vi "FK 5-bar Mechanism.vi"(3 "error in (no error)":errorcluster, 4 "motors angles":dbl[](array[numeric])=[0.0, 0.0, 0.0, 0.0, 0.0, 0.0, 0.0], 5 "Finger in":refnum<class "Finger.lvclass">) -> (0 "error out":errorcluster, 1 "joint angles":dbl[](array[numeric]), 2 "Finger out":refnum<class "Finger.lvclass">)   [LabVIEW 2013, in "Finger.lvclass"]
uses:
  Finger.lvclass
  Finger.lvclass/Finger.ctl
panel:
  out "alpha":dbl
  out "theta":dbl
  out "psi":dbl
  out "phi":dbl
  out "d":dbl
  out "L4":dbl
  out "L3":dbl
  out "L2":dbl
  out "L1":dbl
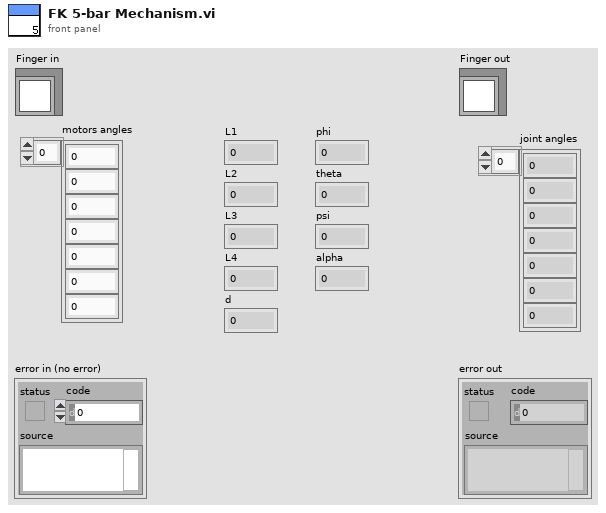
[diagram p1: front panel]
types:
  T1 = typedef "5-bar Side.ctl" = enum16{"Left", "Right"}
  T2 = cluster{"L1":dbl, "L2":dbl, "L3":dbl, "L4":dbl, "d":dbl, "d6":dbl}
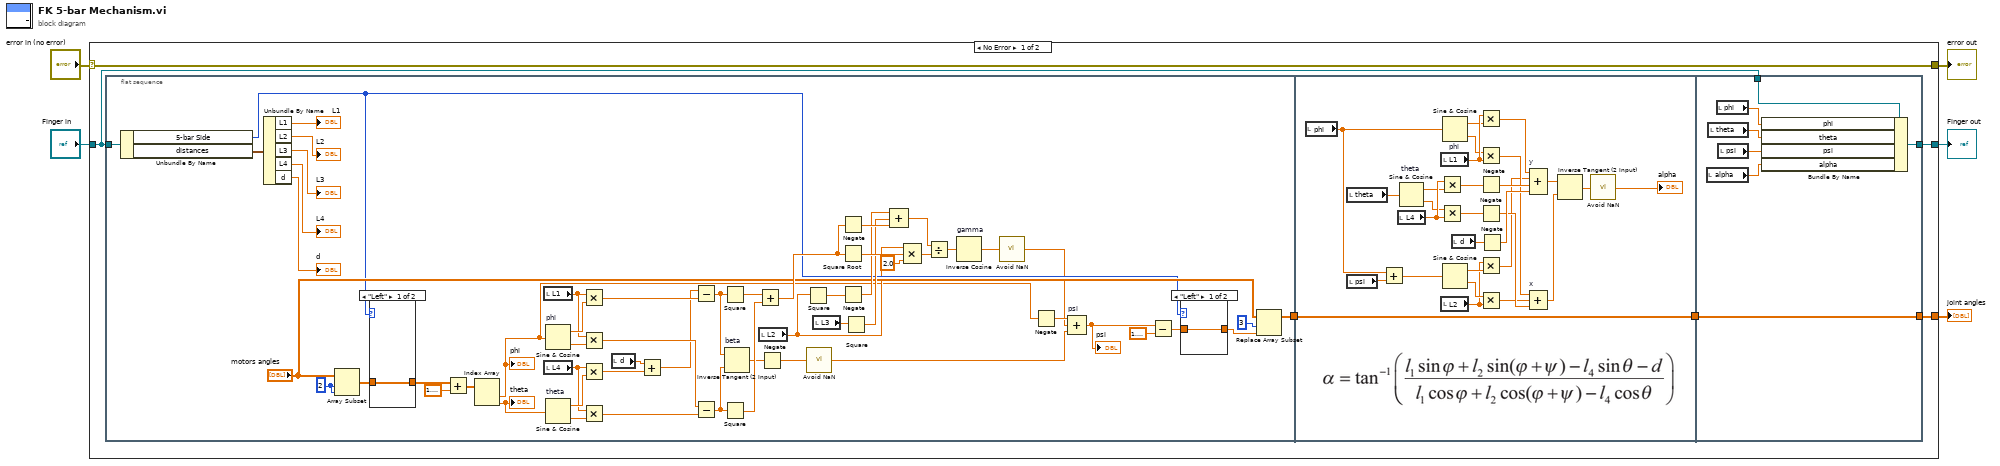
[diagram p0: block diagram]
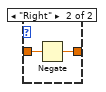
[diagram p2: hidden frame]
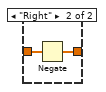
[diagram p3: hidden frame]
diagram:
  n1 = case shown="No Error" "error in (no error)" {
    selector: "error in (no error)" -> [w11 w110]
    tunnel: [w11 w110] -> w4
    tunnel: "Finger in" -> [w6 w109]
    tunnel: [w7 w109] -> w2
    tunnel: [w10 _] -> w1
    frame No Error {
      n2 = flat-sequence {
        tunnel: w6 -> [w31]
        tunnel: [w17] -> w9
        tunnel: w9 -> [w101]
        tunnel: [w101] -> w8
        tunnel: [w108] -> w10
        tunnel: w8 -> [w108]
        tunnel: [w103] -> w7
        tunnel: w6 -> [w102]
        frame #0 {
          w66 = 2 ("index")
          n3 = Unbundle By Name(w31) -> ("5-bar Side"=w30:T1, "distances"=w33:T2)
          n4 = Unbundle By Name(w33) -> ("L1"=→"L1":dbl, "L2"=→"L2":dbl, "L3"=→"L3":dbl, "L4"=→"L4":dbl, "d"=→"d":dbl)
          n5 = Array Subset(array="motors angles", index=w66, length=w66) -> (w35:dbl[])
          n6 = case shown="\"Left\"" w30 {
            tunnel: w35 -> [w71 w73]
            tunnel: [w71 w72] -> w34
            frame "Left" {
            }
            frame "Right" {
              n7 = Negate(x=w73) -> (-x=w72:dbl[])
            }
          }
          n8 = Add(x=w34, y=1.5707963267948966) -> (x+y=w36:dbl[])
          n9 = Index Array(array=w36) -> (element #1=w18:dbl, element #2=w19:dbl)  [unwired: 2 in]
          "phi" <- w18
          "theta" <- w19
          n10 = local read "L1"() -> (w27:dbl)
          n11 = local read "L4"() -> (w24:dbl)
          n12 = Sine & Cosine "phi"(0:w18) -> (1:w29:dbl, 2:w63:dbl)
          n13 = Sine & Cosine "theta"(0:w19) -> (1:w65:dbl, 2:w64:dbl)
          n14 = Multiply(x=w27, y=w29) -> (x*y=w42:dbl)
          n15 = Multiply(x=w27, y=w63) -> (x*y=w61:dbl)
          n16 = Multiply(x=w24, y=w65) -> (x*y=w41:dbl)
          n17 = Multiply(x=w24, y=w64) -> (x*y=w62:dbl)
          n18 = local read "d"() -> (w23:dbl)
          n19 = Add(x=w23, y=w41) -> (x+y=w40:dbl)
          n20 = Subtract(x=w40, y=w42) -> (x-y=w44:dbl)
          n21 = Subtract(x=w61, y=w62) -> (x-y=w43:dbl)
          n22 = Square(x=w44) -> (x^2=w60:dbl)
          n23 = Square(x=w43) -> (x^2=w59:dbl)
          n24 = Inverse Tangent (2 Input) "beta"(1:w43, 2:w44) -> (0:w48:dbl)
          n25 = Add(x=w60, y=w59) -> (x+y=w55:dbl)
          n26 = local read "L2"() -> (w28:dbl)
          n27 = Negate(x=w48) -> (-x=w16:dbl)
          n28 = Square(x=w28) -> (x^2=w57:dbl)
          n29 = call "Avoid NaN.vi"("Value"=w16) -> ("Number"=w15:dbl)
          n30 = local read "L3"() -> (w25:dbl)
          n31 = Negate(x=w55) -> (-x=w58:dbl)
          n32 = Square Root(x=w55) -> (sqrt(x)=w54:dbl)
          n33 = Negate(x=w57) -> (-x=w51:dbl)
          n34 = Square(x=w25) -> (x^2=w50:dbl)
          n35 = Compound Arithmetic op=ADD(w51, w50, w58) -> (w56:dbl)
          n36 = Compound Arithmetic op=MULTIPLY(w28, w54, 2.0 ("value")) -> (w52:dbl)
          n37 = Divide(x=w56, y=w52) -> (x/y=w49:dbl)
          n38 = Inverse Cosine "gamma"(1:w49) -> (0:w14:dbl)
          n39 = call "Avoid NaN.vi"("Value"=w14) -> ("Number"=w13:dbl)
          n40 = Negate(x=w18) -> (-x=w47:dbl)
          n41 = Compound Arithmetic op=ADD "psi"(w47, w13, w15) -> (w12:dbl)
          "psi" <- w12
          n42 = Subtract(x=w12, y=1.5707963267948966) -> (x-y=w37:dbl)
          n43 = case shown="\"Left\"" w30 {
            tunnel: w37 -> [w68 w70]
            tunnel: [w68 w69] -> w39
            frame "Left" {
            }
            frame "Right" {
              n44 = Negate(x=w70) -> (-x=w69:dbl)
            }
          }
          n45 = Replace Array Subset(array="motors angles", new element=w39, index=3) -> (w17:dbl[])
        }
        frame #1 {
          n46 = local read "phi"() -> (w82:dbl)
          n47 = local read "theta"() -> (w87:dbl)
          n48 = local read "psi"() -> (w83:dbl)
          n49 = Add(x=w82, y=w83) -> (x+y=w81:dbl)
          n50 = local read "L4"() -> (w93:dbl)
          n51 = Sine & Cosine "theta"(0:w87) -> (1:w91:dbl, 2:w92:dbl)
          n52 = Multiply(x=w93, y=w91) -> (x*y=w94:dbl)
          n53 = Multiply(x=w92, y=w93) -> (x*y=w97:dbl)
          n54 = local read "L1"() -> (w90:dbl)
          n55 = local read "L2"() -> (w78:dbl)
          n56 = Sine & Cosine "phi"(0:w82) -> (1:w88:dbl, 2:w89:dbl)
          n57 = Sine & Cosine(0:w81) -> (1:w79:dbl, 2:w80:dbl)
          n58 = local read "d"() -> (w100:dbl)
          n59 = Multiply(x=w90, y=w88) -> (x*y=w96:dbl)
          n60 = Multiply(x=w89, y=w90) -> (x*y=w84:dbl)
          n61 = Negate(x=w94) -> (-x=w95:dbl)
          n62 = Negate(x=w97) -> (-x=w98:dbl)
          n63 = Multiply(x=w78, y=w79) -> (x*y=w77:dbl)
          n64 = Multiply(x=w80, y=w78) -> (x*y=w76:dbl)
          n65 = Negate(x=w100) -> (-x=w99:dbl)
          n66 = Compound Arithmetic op=ADD "y"(w96, w77, w95, w99) -> (w85:dbl)
          n67 = Compound Arithmetic op=ADD "x"(w84, w76, w98) -> (w86:dbl)
          n68 = Inverse Tangent (2 Input)(1:w86, 2:w85) -> (0:w75:dbl)
          n69 = call "Avoid NaN.vi"("Value"=w75) -> ("Number"=→"alpha":dbl)
        }
        frame #2 {
          n70 = local read "alpha"() -> (w107:dbl)
          n71 = local read "theta"() -> (w105:dbl)
          n72 = local read "phi"() -> (w104:dbl)
          n73 = local read "psi"() -> (w106:dbl)
          n74 = Bundle By Name(cluster=w102, "phi"=w104, "theta"=w105, "psi"=w106, "alpha"=w107) -> (w103:refnum<class "Finger.lvclass">)
        }
      }
    }
    frame Error {
    }
  }
  "error out" <- w4
  "Finger out" <- w2
  "joint angles" <- w1
